vi "Calib IAS.vi"(7 "Mean Dimension":dbl format="%#_13g", 8 "x 4":dbl, 9 "x 3":dbl, 10 "x 2":dbl, 11 "x":dbl) -> (0 "y 4":dbl, 1 "y 3":dbl, 2 "y 2":dbl, 3 "y 1":dbl)   [LabVIEW 2017]
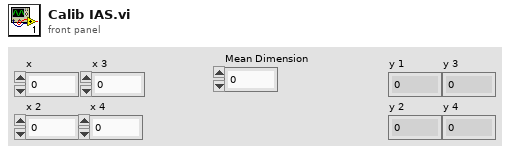
[diagram p1: front panel]
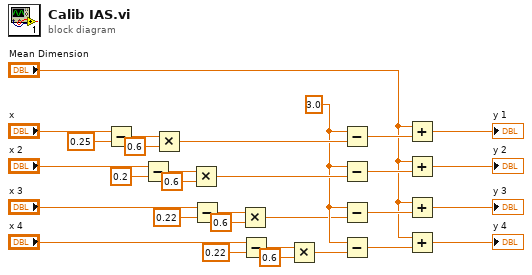
[diagram p0: block diagram]
diagram:
  w10 = 3.0 ("y")
  n1 = Subtract(x="x", y=0.25) -> (x-y=w29:dbl)
  n2 = Subtract(x="x 2", y=0.2) -> (x-y=w26:dbl)
  n3 = Multiply(x=w29, y=0.6) -> (x*y=w14:dbl)
  n4 = Multiply(x=w26, y=0.6) -> (x*y=w12:dbl)
  n5 = Subtract(x="x 3", y=0.22) -> (x-y=w23:dbl)
  n6 = Multiply(x=w23, y=0.6) -> (x*y=w8:dbl)
  n7 = Subtract(x="x 4", y=0.22) -> (x-y=w20:dbl)
  n8 = Multiply(x=w20, y=0.6) -> (x*y=w6:dbl)
  n9 = Subtract(x=w10, y=w14) -> (x-y=w13:dbl)
  n10 = Subtract(x=w10, y=w12) -> (x-y=w11:dbl)
  n11 = Subtract(x=w10, y=w8) -> (x-y=w9:dbl)
  n12 = Subtract(x=w10, y=w6) -> (x-y=w7:dbl)
  n13 = Add(x="Mean Dimension", y=w13) -> (x+y=→"y 1":dbl)
  n14 = Add(x="Mean Dimension", y=w11) -> (x+y=→"y 2":dbl)
  n15 = Add(x="Mean Dimension", y=w9) -> (x+y=→"y 3":dbl)
  n16 = Add(x="Mean Dimension", y=w7) -> (x+y=→"y 4":dbl)
